vi "xy to x y.vi"(11 "Ordered Pairs":T1) -> (0 "Y":dbl[](array[numeric]), 3 "X":dbl[](array[numeric]))   [LabVIEW 2012]
uses:
  <vilib>/Analysis/Matrix/Datatypes/RealMatrix.ctl
  <vilib>/Analysis/Matrix/Numeric/Conversions/Matrix To Array - RM.vi
  <vilib>/Analysis/Matrix/NI_Matrix.lvlib
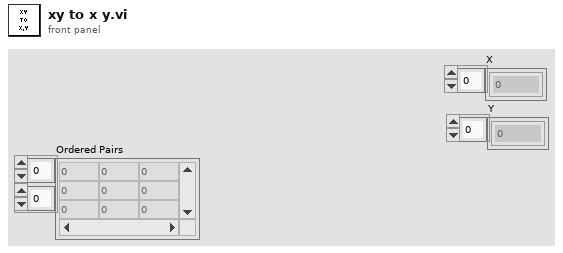
[diagram p1: front panel]
types:
  T1 = typedef "NI_Matrix.lvlib/RealMatrix.ctl" = dbl[][]
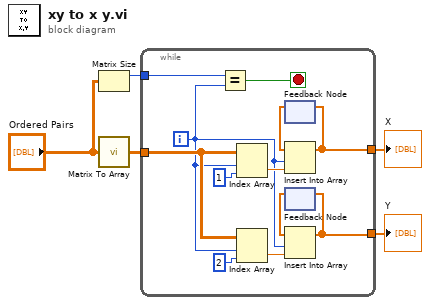
[diagram p0: block diagram]
diagram:
  n1 = Matrix Size(0:"Ordered Pairs") -> (1:w3:i32)  [unwired: 1 out]
  n2 = call-poly <vilib>:"Matrix To Array.vi"("Real Matrix"="Ordered Pairs") -> ("Real 2D Array"=w4:dbl[][])
  n3 = while {
    tunnel: w4 -> [w17]
    tunnel: w3 -> [w16]
    tunnel: [w10] -> w2
    tunnel: [w6] -> w1
    i -> [w7]
    stop <- w15 stop-if-true
    n4 = Equal?(x=w16, y=w7) -> (x = y?=w15:bool)
    n5 = Index Array(array=w17, index (row)=w7, index (col)=1) -> (element=w12:dbl)
    n6 = Index Array(array=w17, index (row)=w7, index (col)=2) -> (element=w8:dbl)
    n7 = feedback #1() -> (w11:dbl[])  [unwired: 1 in]
    n8 = Insert Into Array(array=w11, index=w7, new element=w12) -> (w10:dbl[])
    n9 = feedback-in #1(w10) -> ()
    n10 = feedback #2() -> (w9:dbl[])  [unwired: 1 in]
    n11 = Insert Into Array(array=w9, index=w7, new element=w8) -> (w6:dbl[])
    n12 = feedback-in #2(w6) -> ()
  }
  "X" <- w2
  "Y" <- w1
